vi "XNET Session Property Node.vi"   [LabVIEW 2018]
doc: "Property node used to read/write properties for an XNET Session I/O name."
uses:
  <resource>/objmgr/xnet.rc
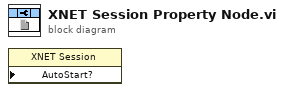
[diagram p0: block diagram]
diagram:
  n1 = property class="XNET Session" props=["AutoStart?"]() -> ()  [unwired: 3 in, 2 out]
